vi "校准流程.vi"(0 "校准模式":T3(ring), 5 "参数下拉列表":u16(ring) items=["CODMn"=21], 7 "测量模式":T1(ring), 9 "量程下拉列表":enum16{"低量程", "高量程"}(ring), 11 "曲线模型":T2={"标液浓度1"=0.0, "测量吸光度1"=0.0, "样品1启用"=FALSE, "标液浓度2"=0.0, "测量吸光度2"=0.0, "样品2启用"=FALSE, "标液浓度3"=0.0, "测量吸光度3"=0.0, "样品3启用"=FALSE, "标液浓度4"=0.0, "测量吸光度4"=0.0, "样品4启用"=FALSE, "标液浓度5"=0.0, "测量吸光度5"=0.0, "样品5启用"=FALSE, "模型"=enum."线性", "精度"=4.0, "XY图"=[], "拟合公式"="", "r^2"=0.0, "标样一校准时间"=timestamp(0 s since 1904-01-01), "标样二校准时间"=timestamp(0 s since 1904-01-01), "标样三校准时间"=timestamp(0 s since 1904-01-01), "标样四校准时间"=timestamp(0 s since 1904-01-01), "标样五校准时间"=timestamp(0 s since 1904-01-01), "二次方程"={"c"=0.0, "x"=0.0, "x^2"=0.0}, "标定时间"=timestamp(0 s since 1904-01-01), "拟合公式 2"="", "r^2 2"=0.0} {"r^2 2" format="%.7f"; "标定时间" format="%<%m/%d/%y %H:%M:%S>T"; "标样五校准时间" format="%<%m/%d/%y %H:%M:%S>T"; "标样四校准时间" format="%<%m/%d/%y %H:%M:%S>T"; "标样三校准时间" format="%<%m/%d/%y %H:%M:%S>T"; "标样二校准时间" format="%<%m/%d/%y %H:%M:%S>T"; "标样一校准时间" format="%<%m/%d/%y %H:%M:%S>T"; "r^2" format="%.7f"; "测量吸光度5" format="%#.6f"; "测量吸光度4" format="%#.6f"; "测量吸光度3" format="%#.6f"; "测量吸光度2" format="%#.6f"; "测量吸光度1" format="%#.6f"}) -> ()   [LabVIEW 2016]
panel:
  out "输出簇":cluster{"数据时间":timestamp, "X值":sgl}
  # "校准时间"
  # "标液浓度"
  # "吸光值显示"
  # "标液一"
  # "标液二"
  # "标液三"
  # "零点"
  # "跨度"
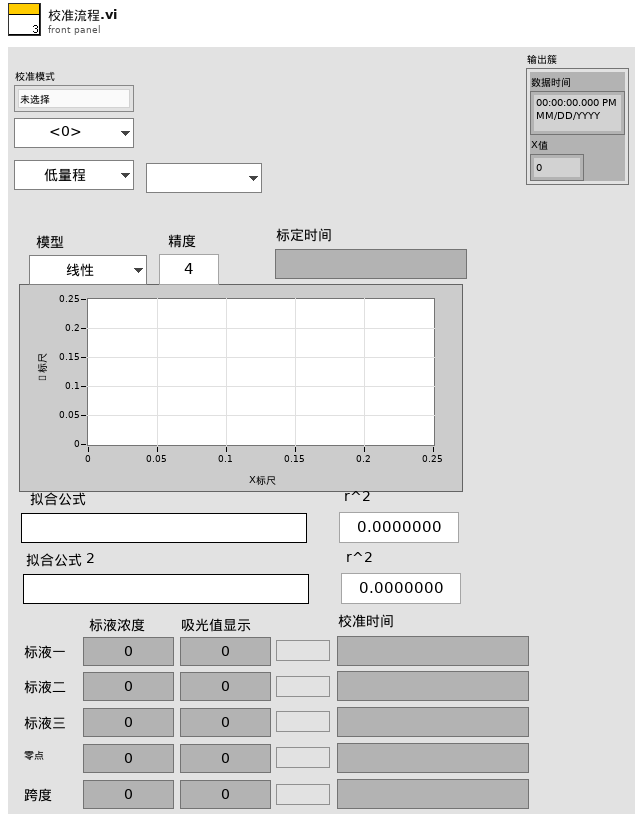
[diagram p1: front panel]
types:
  T1 = enum16{"", "水样测量", "标样核查", "零点核查", "跨度核查", "空白测试", "平行样测试", "加标回收"}
  T2 = cluster{"标液浓度1":dbl, "测量吸光度1":dbl, "样品1启用":bool, "标液浓度2":dbl, "测量吸光度2":dbl, "样品2启用":bool, "标液浓度3":dbl, "测量吸光度3":dbl, "样品3启用":bool, "标液浓度4":dbl, "测量吸光度4":dbl, "样品4启用":bool, "标液浓度5":dbl, "测量吸光度5":dbl, "样品5启用":bool, "模型":enum32{"线性", "多项式", "折线"}, "精度":dbl, "XY图":cluster{"X Values":dbl[], "Y Values":dbl[]}[], "拟合公式":string, "r^2":dbl, "标样一校准时间":timestamp, "标样二校准时间":timestamp, "标样三校准时间":timestamp, "标样四校准时间":timestamp, "标样五校准时间":timestamp, "二次方程":cluster{"c":dbl, "x":dbl, "x^2":dbl}, "标定时间":timestamp, "拟合公式 2":string, "r^2 2":dbl}
  T3 = enum32{"未选择", "空白校准", "标样校准", "标样核查", "零点核查", "跨度核查"}
  T4 = enum16{"初始化", "校准启动", "校准运行中", "测试结束", "获取校准数据", "填充校准数据", "流程结束"}
  T5 = cluster{"站号":u16, "量程切换":enum32{"H", "L", "AUTO"}, "控制命令":u16, "模式设置":enum16{"待机", "连续模式", "周期模式", "定点模式", "受控模式", "手动模式"}, "测量间隔":u16}
  T6 = cluster{"因子编码":u32, "单位":u16, "标样2参考值":sgl, "水样数据时间":timestamp, "水样实测值":sgl, "水样数据标识":string, "标样2数据时间":timestamp, "标样2实测值":sgl, "标样2数据标识":string, "空白数据时间":timestamp, "空白实测值":sgl, "空白数据标识":string, "零点核查数据时间":timestamp, "零点核查实测值":sgl, "零点核查数据标识":string, "跨度核查数据时间":timestamp, "跨度核查实测值":sgl, "跨度核查数据标识":string, "加标回收数据时间":timestamp, "加标回收实测值":sgl, "加标回收数据标识":string, "平行样数据时间":timestamp, "平行样实测值":sgl, "平行样数据标识":string, "标样1参考值":sgl, "标样1数据时间":timestamp, "标样1实测值":sgl, "标样1数据标识":string, "标样核查数据时间":timestamp, "标样核查实测值":sgl, "标样核查数据标识":string}
  T7 = cluster{"系统时间":timestamp, "工作状态":u16, "测量模式":enum16{"待机", "连续模式", "周期模式", "定点模式", "受控模式", "手动模式"}, "告警代码":u16, "故障代码":u16, "日志代码":u16, "软件版本":u16, "测量间隔":u16, "消解实时温度":dbl, "校准间隔（天）":u16, "校准间隔（时）":u16, "周期测量时间（23_16）":u16, "周期测量时间（15_0）":u16, "清洗周期（次数）":u16, "运行模式":u16, "自动校准状态":u16, "自动清洗状态":u16}
  T8 = cluster{"标液浓度1":dbl, "测量吸光度1":dbl, "样品1启用":bool, "标液浓度2":dbl, "测量吸光度2":dbl, "样品2启用":bool, "标液浓度3":dbl, "测量吸光度3":dbl, "样品3启用":bool, "标液浓度4":dbl, "测量吸光度4":dbl, "样品4启用":bool, "标液浓度5":dbl, "测量吸光度5":dbl, "样品5启用":bool, "模型":enum32{"线性", "多项式", "折线"}, "精度":dbl, "XY图":cluster{"X Values":dbl[], "Y Values":dbl[]}[], "拟合公式":string, "r^2":dbl, "标样一校准时间":timestamp, "标样二校准时间":timestamp, "标样三校准时间":timestamp, "标样四校准时间":timestamp, "标样五校准时间":timestamp, "二次方程":cluster{"c":dbl, "x":dbl, "x^2":dbl}, "标定时间":timestamp, "拟合公式 2":string, "r^2 2":dbl}[][]
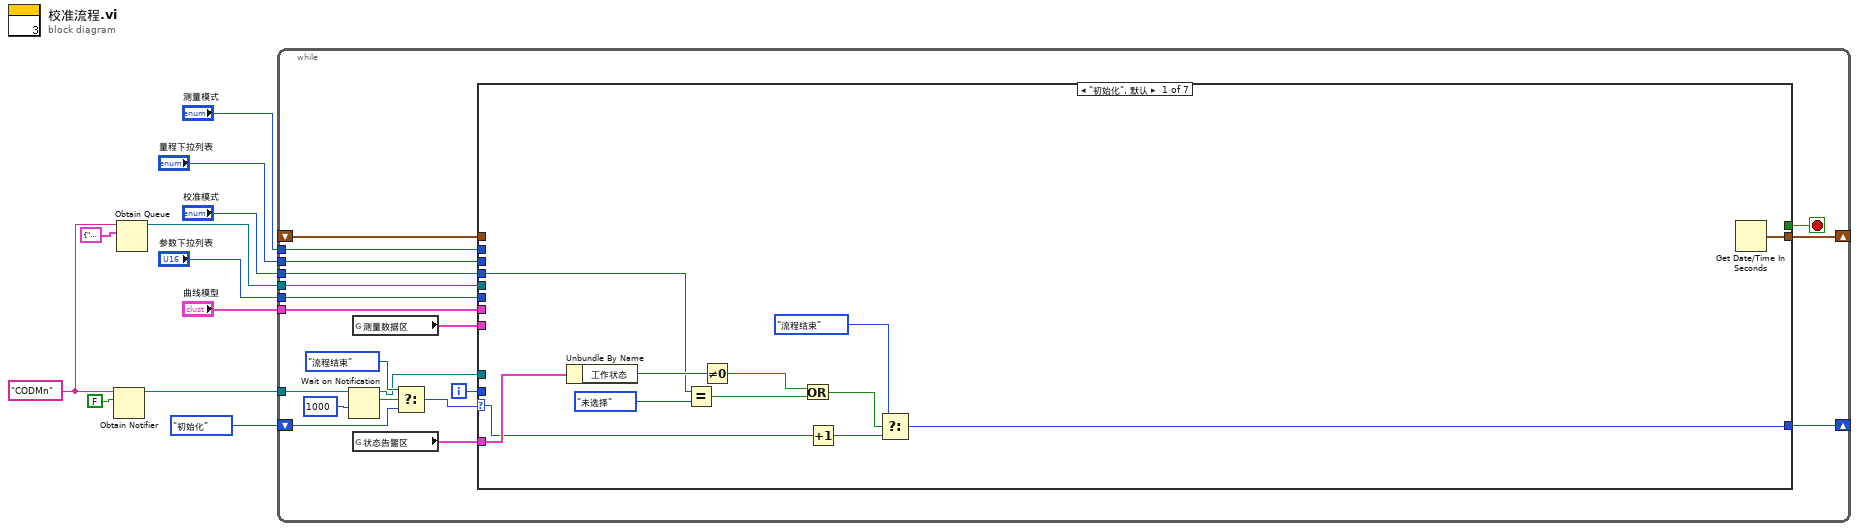
[diagram p0: block diagram]
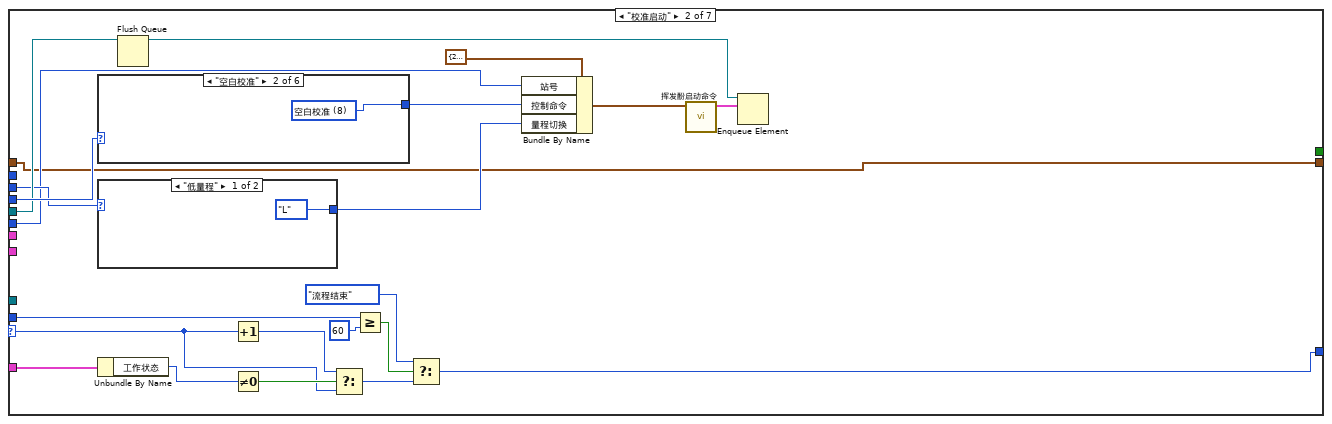
[diagram p2: hidden frame]
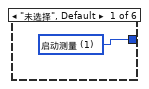
[diagram p3: hidden frame]
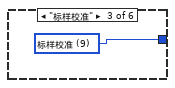
[diagram p4: hidden frame]
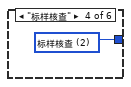
[diagram p5: hidden frame]
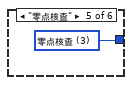
[diagram p6: hidden frame]
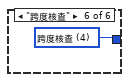
[diagram p7: hidden frame]
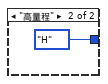
[diagram p8: hidden frame]
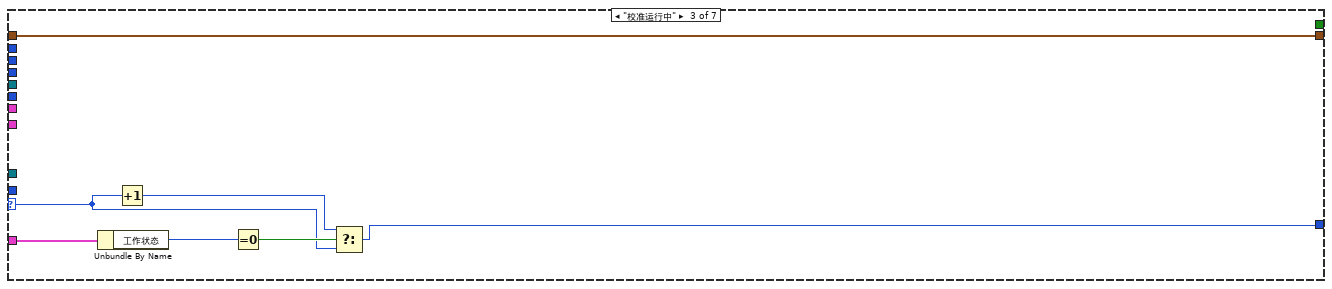
[diagram p9: hidden frame]
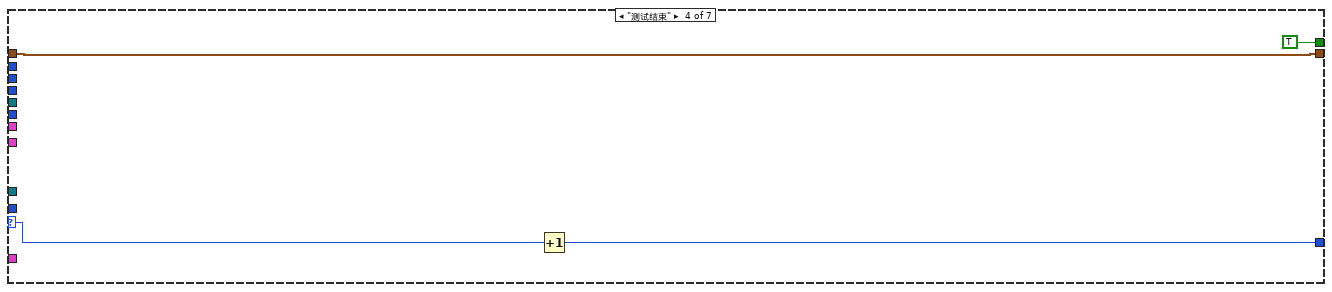
[diagram p10: hidden frame]
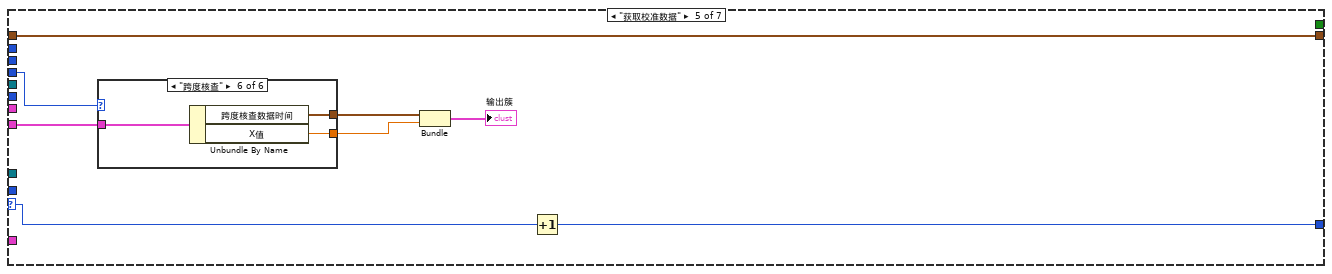
[diagram p11: hidden frame]
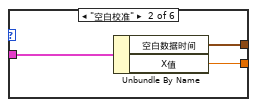
[diagram p13: hidden frame]
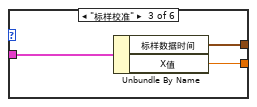
[diagram p14: hidden frame]
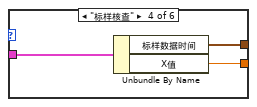
[diagram p15: hidden frame]
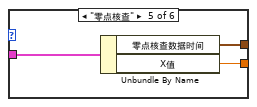
[diagram p16: hidden frame]
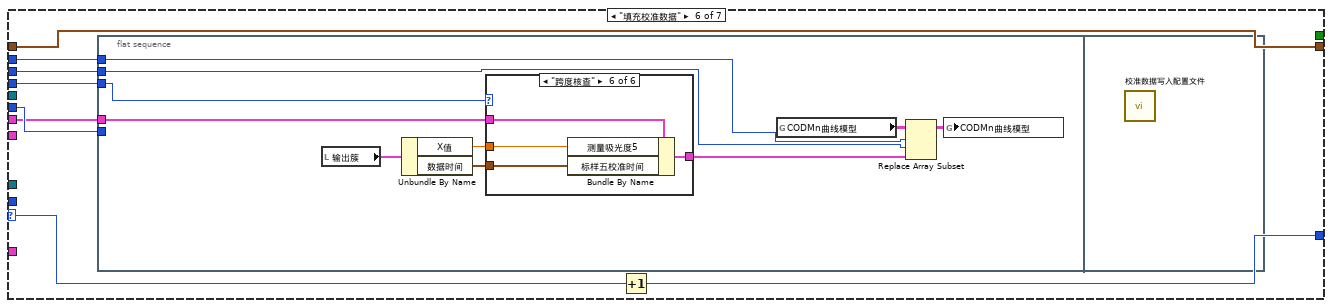
[diagram p17: hidden frame]
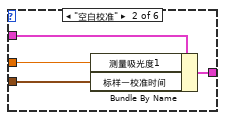
[diagram p19: hidden frame]
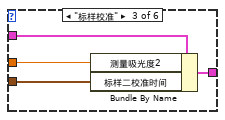
[diagram p20: hidden frame]
diagram:
  w1 = "CODMn" ("名称（未命名）")
  n1 = Obtain Notifier(name (unnamed)=w1, notification data type=FALSE) -> (notifier out=w2:refnum<notifier>)  [unwired: 2 in, 2 out]
  n2 = Obtain Queue(name (unnamed)=w1, element data type=cluster{"命令":string, "data":variant} {"命令"="", "data"=variant}) -> (queue out=w8:refnum<queue>)  [unwired: 3 in, 2 out]
  n3 = while {
    tunnel: "校准模式" -> [w30]
    shift-right: [w28] -> _
    shift-left: T4."初始化" ("枚举") -> [w15]
    tunnel: w8 -> [w31]
    tunnel: "量程下拉列表" -> [w27]
    tunnel: "参数下拉列表" -> [w26]
    shift-right: [w25] -> _
    shift-left: _ -> [w24]
    tunnel: "曲线模型" -> [w21]
    tunnel: "测量模式" -> [w20]
    tunnel: w2 -> [w18]
    i -> [w19]
    stop <- w29 stop-if-true
    n4 = Wait on Notification(notifier=w18, timeout in ms (-1)=1000 ("超时毫秒(-1)")) -> (notifier out=w13:refnum<notifier>, notification=w16:bool)  [unwired: 2 in, 2 out]
    n5 = global read "VAR挥发酚全局变量.vi" "测量数据区"() -> (w23:T6)
    n6 = global read "VAR挥发酚全局变量.vi" "状态告警区"() -> (w22:T7)
    n7 = Select(t=T4."流程结束", s=w16, f=w15) -> (s? t:f=w12:T4)
    n8 = case shown="\"初始化\", 默认" w12 {
      selector: w12 -> [w39 w52 w79 w84 w92 w115 w149]
      tunnel: w31 -> [_ w59 _ _ _ _ w147]
      tunnel: w30 -> [w35 w60 _ _ w89 w109 _]
      tunnel: [_ _ _ TRUE _ _ TRUE] -> w29
      tunnel: [w37 w46 w77 w81 w85 w108 w149] -> w28
      tunnel: w27 -> [_ w58 _ _ _ w112 _]
      tunnel: w26 -> [_ w57 _ _ _ w113 _]
      tunnel: w22 -> [w42 w55 w75 _ _ _ _]
      tunnel: [w43 w56 w76 w83 w91 w114 w148] -> w25
      tunnel: w24 -> [_ w56 w76 w83 w91 w114 w148]
      tunnel: w23 -> [_ _ _ _ w90 _ _]
      tunnel: w21 -> [_ _ _ _ _ w111 _]
      tunnel: w20 -> [_ _ _ _ _ w110 _]
      tunnel: w19 -> [_ w50 _ _ _ _ _]
      tunnel: w13 -> [_ _ _ _ _ _ w146]
      frame "初始化", Default {
        n9 = Unbundle By Name(w42) -> ("工作状态"=w41:u16)
        n10 = Equal?(x=w35, y=T3."未选择") -> (x = y?=w32:bool)
        n11 = Not Equal To 0?(x=w41) -> (x != 0?=w40:bool)
        n12 = Or(x=w40, y=w32) -> (x .or. y?=w33:bool)
        n13 = Increment(x=w39) -> (x+1=w38:T4)
        n14 = Select(t=T4."流程结束", s=w33, f=w38) -> (s? t:f=w37:T4)
        n15 = Get Date/Time In Seconds() -> (seconds since 1Jan1904=w43:timestamp)
      }
      frame "校准启动" {
        n16 = case shown="\"空白校准\"" w60 {
          tunnel: [w66 w67 w68 w69 w70 w71] -> w65
          frame "未选择", Default {
            w66 = u16 1 items=["启动测量"=1, "标样核查"=2, "零点核查"=3, "跨度核查"=4, "空白测试"=5, "平行样测试"=6, "加标回收"=7, "空白校准"=8, "标样校准"=9, "初始化（清洗）"=10, "停止测试"=11, "仪器重启"=12, "校时"=13, "模式设置"=14, "测量间隔设置"=15, "调试"=22, "填充管路"=30, "清洗管路"=31, "清洗反应杯"=32] ("控制命令")
          }
          frame "空白校准" {
            w67 = u16 8 items=["启动测量"=1, "标样核查"=2, "零点核查"=3, "跨度核查"=4, "空白测试"=5, "平行样测试"=6, "加标回收"=7, "空白校准"=8, "标样校准"=9, "初始化（清洗）"=10, "停止测试"=11, "仪器重启"=12, "校时"=13, "模式设置"=14, "测量间隔设置"=15, "调试"=22, "填充管路"=30, "清洗管路"=31, "清洗反应杯"=32] ("控制命令")
          }
          frame "标样校准" {
            w68 = u16 9 items=["启动测量"=1, "标样核查"=2, "零点核查"=3, "跨度核查"=4, "空白测试"=5, "平行样测试"=6, "加标回收"=7, "空白校准"=8, "标样校准"=9, "初始化（清洗）"=10, "停止测试"=11, "仪器重启"=12, "校时"=13, "模式设置"=14, "测量间隔设置"=15, "调试"=22, "填充管路"=30, "清洗管路"=31, "清洗反应杯"=32] ("控制命令")
          }
          frame "标样核查" {
            w69 = u16 2 items=["启动测量"=1, "标样核查"=2, "零点核查"=3, "跨度核查"=4, "空白测试"=5, "平行样测试"=6, "加标回收"=7, "空白校准"=8, "标样校准"=9, "初始化（清洗）"=10, "停止测试"=11, "仪器重启"=12, "校时"=13, "模式设置"=14, "测量间隔设置"=15, "调试"=22, "填充管路"=30, "清洗管路"=31, "清洗反应杯"=32] ("控制命令")
          }
          frame "零点核查" {
            w70 = u16 3 items=["启动测量"=1, "标样核查"=2, "零点核查"=3, "跨度核查"=4, "空白测试"=5, "平行样测试"=6, "加标回收"=7, "空白校准"=8, "标样校准"=9, "初始化（清洗）"=10, "停止测试"=11, "仪器重启"=12, "校时"=13, "模式设置"=14, "测量间隔设置"=15, "调试"=22, "填充管路"=30, "清洗管路"=31, "清洗反应杯"=32] ("控制命令")
          }
          frame "跨度核查" {
            w71 = u16 4 items=["启动测量"=1, "标样核查"=2, "零点核查"=3, "跨度核查"=4, "空白测试"=5, "平行样测试"=6, "加标回收"=7, "空白校准"=8, "标样校准"=9, "初始化（清洗）"=10, "停止测试"=11, "仪器重启"=12, "校时"=13, "模式设置"=14, "测量间隔设置"=15, "调试"=22, "填充管路"=30, "清洗管路"=31, "清洗反应杯"=32] ("控制命令")
          }
        }
        n17 = case shown="\"低量程\"" w58 {
          tunnel: [enum32{"H", "L", "AUTO"}."L" ("量程切换") enum32{"H", "L", "AUTO"}."H" ("量程切换")] -> w64
          frame "低量程" {
          }
          frame "高量程" {
          }
        }
        n18 = Unbundle By Name(w55) -> ("工作状态"=w54:u16)
        n19 = Flush Queue(queue=w59) -> (queue out=w62:refnum<queue>)  [unwired: 1 in, 2 out]
        n20 = Increment(x=w52) -> (x+1=w51:T4)
        n21 = Not Equal To 0?(x=w54) -> (x != 0?=w53:bool)
        n22 = Select(t=w51, s=w53, f=w52) -> (s? t:f=w47:T4)
        n23 = Greater Or Equal?(x=w50, y=60) -> (x >= y?=w48:bool)
        n24 = Select(t=T4."流程结束", s=w48, f=w47) -> (s? t:f=w46:T4)
        n25 = Bundle By Name(cluster=T5 {"站号"=21, "量程切换"=enum."AUTO", "控制命令"=0, "模式设置"=enum."待机", "测量间隔"=0} ("参数"), "站号"=w57, "控制命令"=w65, "量程切换"=w64) -> (w63:T5)
        n26 = call "挥发酚启动命令.vi"("参数"=w63) -> ("启动命令"=w61:cluster{"命令":string, "data":variant})  [unwired: 10 in]
        n27 = Enqueue Element(queue=w62, element=w61) -> ()  [unwired: 2 in, 3 out]
      }
      frame "校准运行中" {
        n28 = Unbundle By Name(w75) -> ("工作状态"=w74:u16)
        n29 = Increment(x=w79) -> (x+1=w78:T4)
        n30 = Equal To 0?(x=w74) -> (x = 0?=w80:bool)
        n31 = Select(t=w78, s=w80, f=w79) -> (s? t:f=w77:T4)
      }
      frame "测试结束" {
        n32 = Increment(x=w84) -> (x+1=w81:T4)
      }
      frame "获取校准数据" {
        n33 = case shown="\"跨度核查\"" w89 {
          tunnel: w90 -> [_ w95 w98 w101 w104 w107]
          tunnel: [_ w94 w97 w100 w103 w106] -> w88
          tunnel: [_ w93 w96 w99 w102 w105] -> w87
          frame "未选择", Default {
          }
          frame "空白校准" {
            n34 = Unbundle By Name(w95) -> ("空白数据时间"=w94:timestamp, "X值"=w93:sgl)
          }
          frame "标样校准" {
            n35 = Unbundle By Name(w98) -> ("标样数据时间"=w97:timestamp, "X值"=w96:sgl)
          }
          frame "标样核查" {
            n36 = Unbundle By Name(w101) -> ("标样数据时间"=w100:timestamp, "X值"=w99:sgl)
          }
          frame "零点核查" {
            n37 = Unbundle By Name(w104) -> ("零点核查数据时间"=w103:timestamp, "X值"=w102:sgl)
          }
          frame "跨度核查" {
            n38 = Unbundle By Name(w107) -> ("跨度核查数据时间"=w106:timestamp, "X值"=w105:sgl)
          }
        }
        n39 = Bundle("跨度核查数据时间"=w88, "X值"=w87) -> (→"输出簇":cluster{"跨度核查数据时间":timestamp, "X值":sgl})  [unwired: 1 in]
        n40 = Increment(x=w92) -> (x+1=w85:T4)
      }
      frame "填充校准数据" {
        n41 = flat-sequence {
          tunnel: w113 -> [_]
          tunnel: w112 -> [w125]
          tunnel: w111 -> [w124]
          tunnel: w110 -> [w122]
          tunnel: w109 -> [w121]
          frame #0 {
            n42 = local read "输出簇"() -> (w120:cluster{"数据时间":timestamp, "X值":sgl})
            n43 = Unbundle By Name(w120) -> ("X值"=w119:sgl, "数据时间"=w118:timestamp)
            n44 = case shown="\"跨度核查\"" w121 {
              tunnel: w124 -> [_ w129 w133 w137 w141 w145]
              tunnel: [_ w128 w132 w136 w140 w144] -> w123
              tunnel: w119 -> [_ w127 w131 w135 w139 w143]
              tunnel: w118 -> [_ w126 w130 w134 w138 w142]
              frame "未选择", Default {
              }
              frame "空白校准" {
                n45 = Bundle By Name(cluster=w129, "测量吸光度1"=w127, "标样一校准时间"=w126) -> (w128:T2)
              }
              frame "标样校准" {
                n46 = Bundle By Name(cluster=w133, "测量吸光度2"=w131, "标样二校准时间"=w130) -> (w132:T2)
              }
              frame "标样核查" {
                n47 = Bundle By Name(cluster=w137, "测量吸光度3"=w135, "标样三校准时间"=w134) -> (w136:T2)
              }
              frame "零点核查" {
                n48 = Bundle By Name(cluster=w141, "测量吸光度4"=w139, "标样四校准时间"=w138) -> (w140:T2)
              }
              frame "跨度核查" {
                n49 = Bundle By Name(cluster=w145, "测量吸光度5"=w143, "标样五校准时间"=w142) -> (w144:T2)
              }
            }
            n50 = global read "校准数据全局变量.vi" "CODMn曲线模型"() -> (w117:T8)
            n51 = Replace Array Subset(array=w117, new element=w123, index (row)=w122, index (col)=w125) -> (w116:T8)
            n52 = global write "校准数据全局变量.vi" "CODMn曲线模型"(w116) -> ()
          }
          frame #1 {
            n53 = call "校准数据写入配置文件.vi"() -> ()  [unwired: 11 in, 1 out]
          }
        }
        n54 = Increment(x=w115) -> (x+1=w108:T4)
      }
      frame "流程结束" {
        n55 = Release Notifier(notifier=w146) -> ()  [unwired: 2 in, 3 out]
        n56 = Release Queue(queue=w147) -> ()  [unwired: 2 in, 3 out]
      }
    }
  }
